vi "SyncPIDAdjValue.vi"(0 "NP":dbl(slide) caption="P" scale=0.0..99.0 scale format="%.3f", 1 "NI":dbl(slide) caption="I" scale=0.0..99.0 scale format="%.3f", 2 "refPIDAdj":refnum<vi>, 3 "NPS":T1(ring), 4 "NIS":T1(ring), 5 "ND":dbl(slide) caption="D" scale=0.0..99.0 scale format="%.3f", 8 "NDS":T1(ring)) -> ()   [LabVIEW 2024]
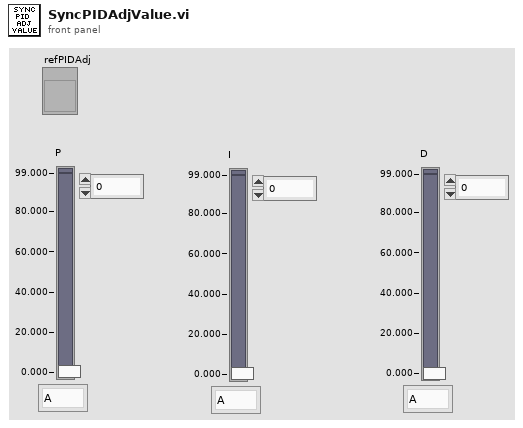
[diagram p1: front panel]
types:
  T1 = enum16{"A", "B", "C", "D", "E", "F", "G", "H", "I"}
  T2 = cluster{"PID Mode":enum16{"Torque", "Speed", "Ramp", "Amp", "Watts In", "Watts Out"}, "NP":dbl, "NI":dbl, "ND":dbl, "NPS":string, "NIS":string, "NDS":string}
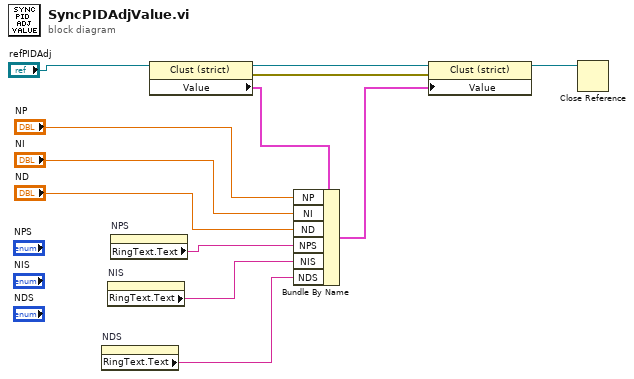
[diagram p0: block diagram]
diagram:
  n1 = property on="NDS" class="Enum (strict)"() -> ("RingText.Text"=w5:string)  [unwired: 2 in, 2 out]
  n2 = property on="NIS" class="Enum (strict)"() -> ("RingText.Text"=w6:string)  [unwired: 2 in, 2 out]
  n3 = property on="NPS" class="Enum (strict)"() -> ("RingText.Text"=w7:string)  [unwired: 2 in, 2 out]
  n4 = property class="Clust (strict)"(reference="refPIDAdj") -> (reference out=w4:refnum<vi>, error out=w3:errorcluster, "Value"=w11:T2)  [unwired: 1 in]
  n5 = Bundle By Name(cluster=w11, "NP"="NP", "NI"="NI", "ND"="ND", "NPS"=w7, "NIS"=w6, "NDS"=w5) -> (w2:T2)
  n6 = property class="Clust (strict)"(reference=w4, error in=w3, "Value"=w2) -> (reference out=w1:refnum<vi>)  [unwired: 1 out]
  n7 = Close Reference(reference=w1) -> ()  [unwired: 1 in, 1 out]
